vi "Update INI File_Prober Control.vi"(0 "configuration file path":path=path "C:/LabVIEW Code/Test Data/Prober Exp/Prober Configuration File .ini", 2 "Test Started":bool, 11 "Error In":errorcluster) -> (15 "Error Out":errorcluster)   [LabVIEW 2013]
uses:
  <vilib>/Utility/config.llb/Write Key (String).vi
  <vilib>/Utility/config.llb/NI_LVConfig.lvlib
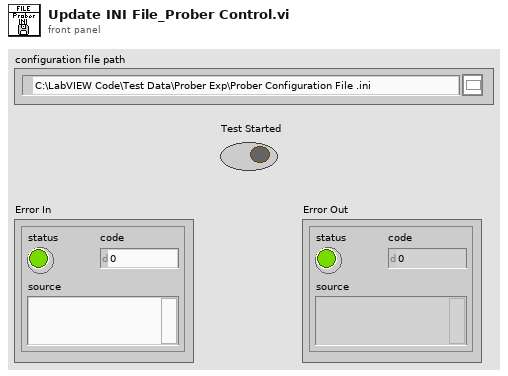
[diagram p1: front panel]
types:
  T1 = typedef "NI_LVConfig.lvlib/Config Data RefNum.ctl" = refnum<k1>
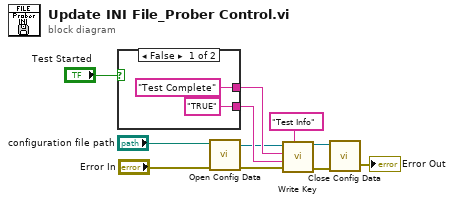
[diagram p0: block diagram]
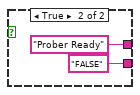
[diagram p2: hidden frame]
diagram:
  n1 = case shown="False" "Test Started" {
    tunnel: ["Test Complete" ("key") "Prober Ready" ("key")] -> w7
    tunnel: ["TRUE" ("key") "FALSE" ("key")] -> w6
    frame False {
    }
    frame True {
    }
  }
  n2 = call <vilib>:"Open Config Data.vi"("error in (no error)"="Error In", "configuration file path"="configuration file path") -> ("error out"=w5:errorcluster, "refnum"=w4:T1)  [unwired: 7 in, 1 out]
  n3 = call-poly <vilib>:"Write Key.vi"("section"="Test Info", "error in (no error)"=w5, "value"=w6, "key"=w7, "refnum"=w4) -> ("error out"=w10:errorcluster, "refnum out"=w9:T1)  [unwired: 4 in, 1 out]
  n4 = call <vilib>:"Close Config Data.vi"("error in (no error)"=w10, "refnum"=w9) -> ("error out"=→"Error Out":errorcluster)  [unwired: 8 in, 1 out]
